vi "Arm Mode Control.vi"(1 "Motor Speed In":dbl, 2 "Current Angle":dbl) -> (0 "Motor Speed Out":dbl)   [LabVIEW 2013]
uses:
  Robot Global Data.vi
panel:
  in  "Shoot Angle Range":dbl=3.0
  in  "Pre-Shoot Angle":dbl=90.0
  in  "Hold Angle":dbl=160.0
  in  "Catch Angle":dbl=145.0
  in  "Pick Up Angle":dbl=90.0
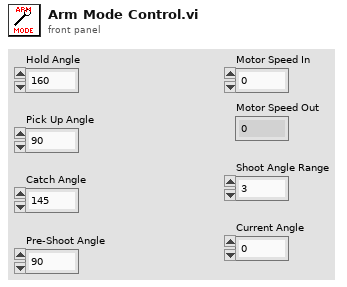
[diagram p1: front panel]
types:
  T1 = enum16{"Hold", "Pick Up", "Catch", "Aim", "Shoot", "Joystick"}
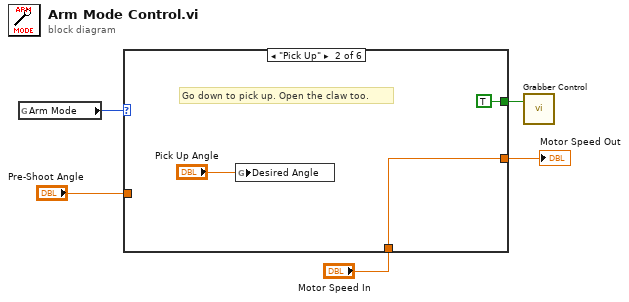
[diagram p0: block diagram]
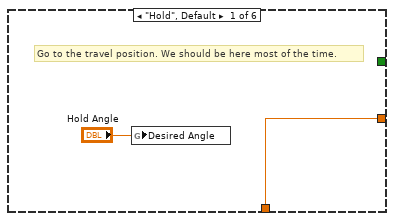
[diagram p2: hidden frame]
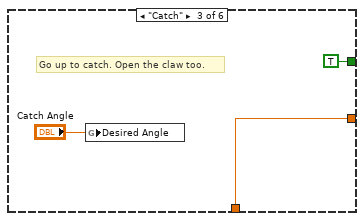
[diagram p3: hidden frame]
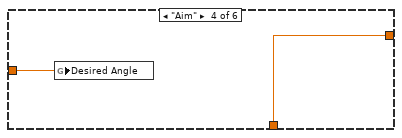
[diagram p4: hidden frame]
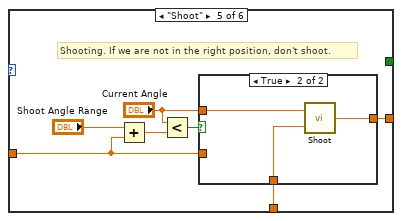
[diagram p5: hidden frame]
diagram:
  n1 = global read "Robot Global Data.vi" "Arm Mode"() -> (w5:T1)
  n2 = case shown="\"Pick Up\"" w5 {
    tunnel: "Motor Speed In" -> [w6 w9 w12 w15 w19 w27]
    tunnel: [w6 w9 w12 w15 w18 w27] -> w3
    tunnel: [_ TRUE TRUE _ _ _] -> w2
    tunnel: "Pre-Shoot Angle" -> [_ _ _ w14 w17 _]
    frame "Hold", Default {
      # "Go to the travel position. We should be here most of the time."
      n3 = global write "Robot Global Data.vi" "Desired Angle"("Hold Angle") -> ()
    }
    frame "Pick Up" {
      # "Go down to pick up. Open the claw too."
      n4 = global write "Robot Global Data.vi" "Desired Angle"("Pick Up Angle") -> ()
    }
    frame "Catch" {
      # "Go up to catch. Open the claw too."
      n5 = global write "Robot Global Data.vi" "Desired Angle"("Catch Angle") -> ()
    }
    frame "Aim" {
      n6 = global write "Robot Global Data.vi" "Desired Angle"(w14) -> ()
    }
    frame "Shoot" {
      # "Shooting. If we are not in the right position, don't shoot."
      n7 = Add(x="Shoot Angle Range", y=w17) -> (x+y=w21:dbl)
      n8 = Less?(x="Current Angle", y=w21) -> (x < y?=w22:bool)
      n9 = case shown="True" w22 {
        tunnel: "Current Angle" -> [_ w26]
        tunnel: w17 -> [_ _]
        tunnel: w19 -> [w23 w25]
        tunnel: [w23 w24] -> w18
        frame False {
        }
        frame True {
          n10 = call "Shoot.vi"("Current Motor SetPoint"=w25, "Current Angle"=w26) -> ("New Motor Setpoint"=w24:dbl)
        }
      }
    }
    frame "Joystick" {
    }
  }
  "Motor Speed Out" <- w3
  n11 = call "Grabber Control.vi"("Holding Button"=w2) -> ()  [unwired: 2 in]
